vi "Reset credit.vi"(8 "error in (no error)":errorcluster, 10 "Compra realizada?":bool, 11 "USD Actor in":refnum<class "USD Actor.lvclass">) -> (0 "error out":errorcluster, 3 "USD Actor out":refnum<class "USD Actor.lvclass">)   [LabVIEW 2020, in "USD Actor.lvlib" / "USD Actor.lvclass"]
uses:
  USD Actor.lvclass
  USD Actor.lvclass/USD Actor.ctl
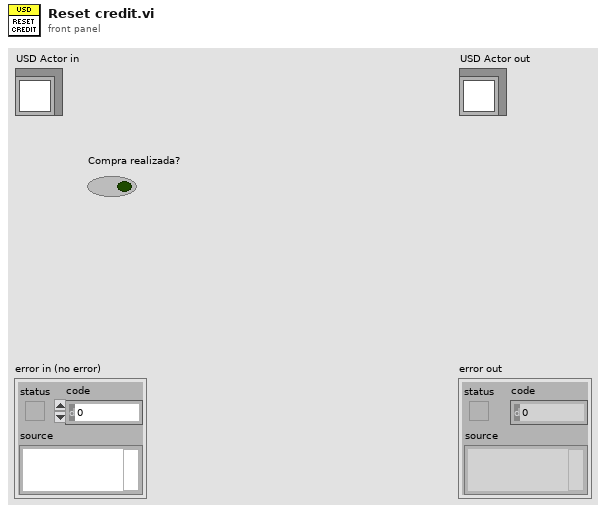
[diagram p1: front panel]
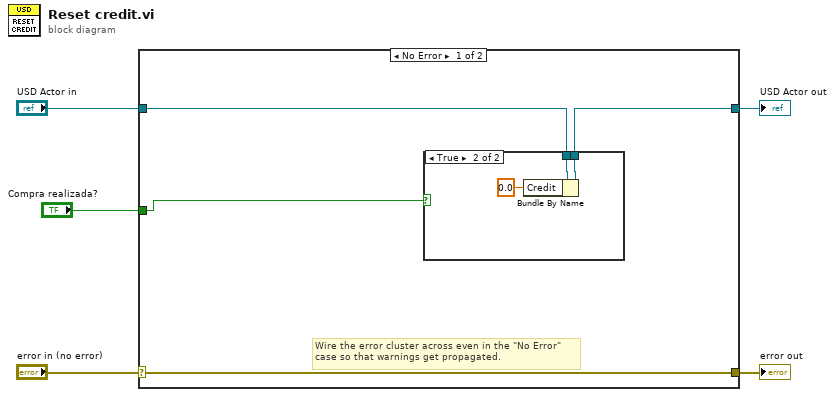
[diagram p0: block diagram]
diagram:
  n1 = case shown="No Error" "error in (no error)" {
    selector: "error in (no error)" -> [w8 w15]
    tunnel: [w8 w15] -> w4
    tunnel: [w7 w14] -> w2
    tunnel: "USD Actor in" -> [w9 w14]
    tunnel: "Compra realizada?" -> [w6 _]
    frame No Error {
      # "Wire the error cluster across even in the \"No Error\"\ncase so that warnings get propagated."
      n2 = case shown="True" w6 {
        tunnel: w9 -> [w10 w13]
        tunnel: [w10 w12] -> w7
        frame False {
        }
        frame True {
          n3 = Bundle By Name(cluster=w13, "Credit"=0.0) -> (w12:refnum<class "USD Actor.lvclass">)
        }
      }
    }
    frame Error {
    }
  }
  "error out" <- w4
  "USD Actor out" <- w2
